vi "graph difference.vi"() -> ()   [LabVIEW 2023]
uses:
  <vilib>/addons/control/pid/autopid.llb/PID autotuning parameters (adv).ctl
  <vilib>/express/express analysis/Spectral/Block/exnSpectralBlock spectral measurements RMS poly.vi
  <vilib>/express/express analysis/Spectral/Block/exnSpectralBlock spectral measurements RMS DDT.vi
  <vilib>/express/express analysis/Spectral/XNode/ExpressSpectralMeasurementsBlockNode.xnode
  <vilib>/measure/NI_MABase.lvlib
  <vilib>/addons/control/pid/NI_PID_autopid.lvlib
panel:
  out "Control":waveform(dbl)(graph)
  in  "Target Frequency":dbl=10.0 caption="Frequency"
  out "tuning completed?":bool
  out "tuned PID gains":T1={"proportional gain (Kc)"=1.0, "integral time (Ti, min)"=0.01, "derivative time (Td, min)"=0.0} {"derivative time (Td, min)" format="%#.6g"; "integral time (Ti, min)" format="%#.6g"; "proportional gain (Kc)" format="%#.6g"}
  in  "Autotune Control":bool
  out "Backward 2":bool
  out "Forward 2":bool
  out "dt":dbl
  out "Target Waveform Graph":dynamicdata(graph)
  out "Fast Fourier Transform Target":dynamicdata(graph)
  out "Frequency Control Array":dbl[](array[numeric])
  in  "Frequency Control":dbl
  in  "amplitude 2":dbl=1.0 format="%0.2p"
  out "Phase 2":dbl
  in  "Frequency 2":dbl
  in  "stop 3":bool
  in  "frequency":dbl=10.0 format="%0.2p"
  out "Waveform Graph 2":waveform(dbl)(graph)
  in  "sampling info 2":cluster{"Fs":dbl, "#s":dbl}={"Fs"=1000.0, "#s"=1000.0} {"Fs" format="%.2p"}
  out "Difference Graph":dynamicdata(graph)
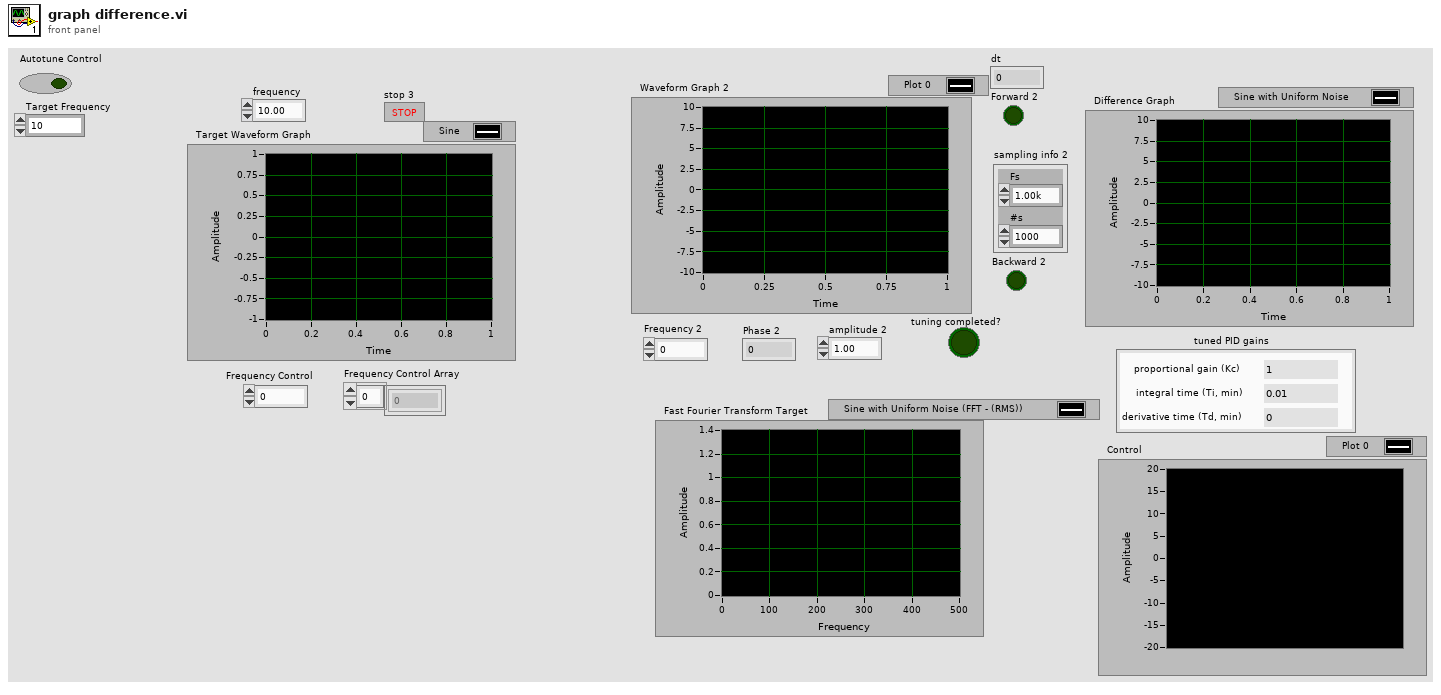
[diagram p1: front panel]
types:
  T1 = cluster{"proportional gain (Kc)":dbl, "integral time (Ti, min)":dbl, "derivative time (Td, min)":dbl}
  T2 = cluster{"averaging mode":u16, "weighting mode":u16, "number of averages":u32}
  T3 = cluster{"dB On (F)":bool, "unwrap phase (F)":bool, "convert to degree (F)":bool}
  T4 = typedef "NI_PID_autopid.lvlib/PID autotuning parameters (adv).ctl" = cluster{"technique":u16, "type of controller":u16, "control specification":u16, "amplitude":dbl}
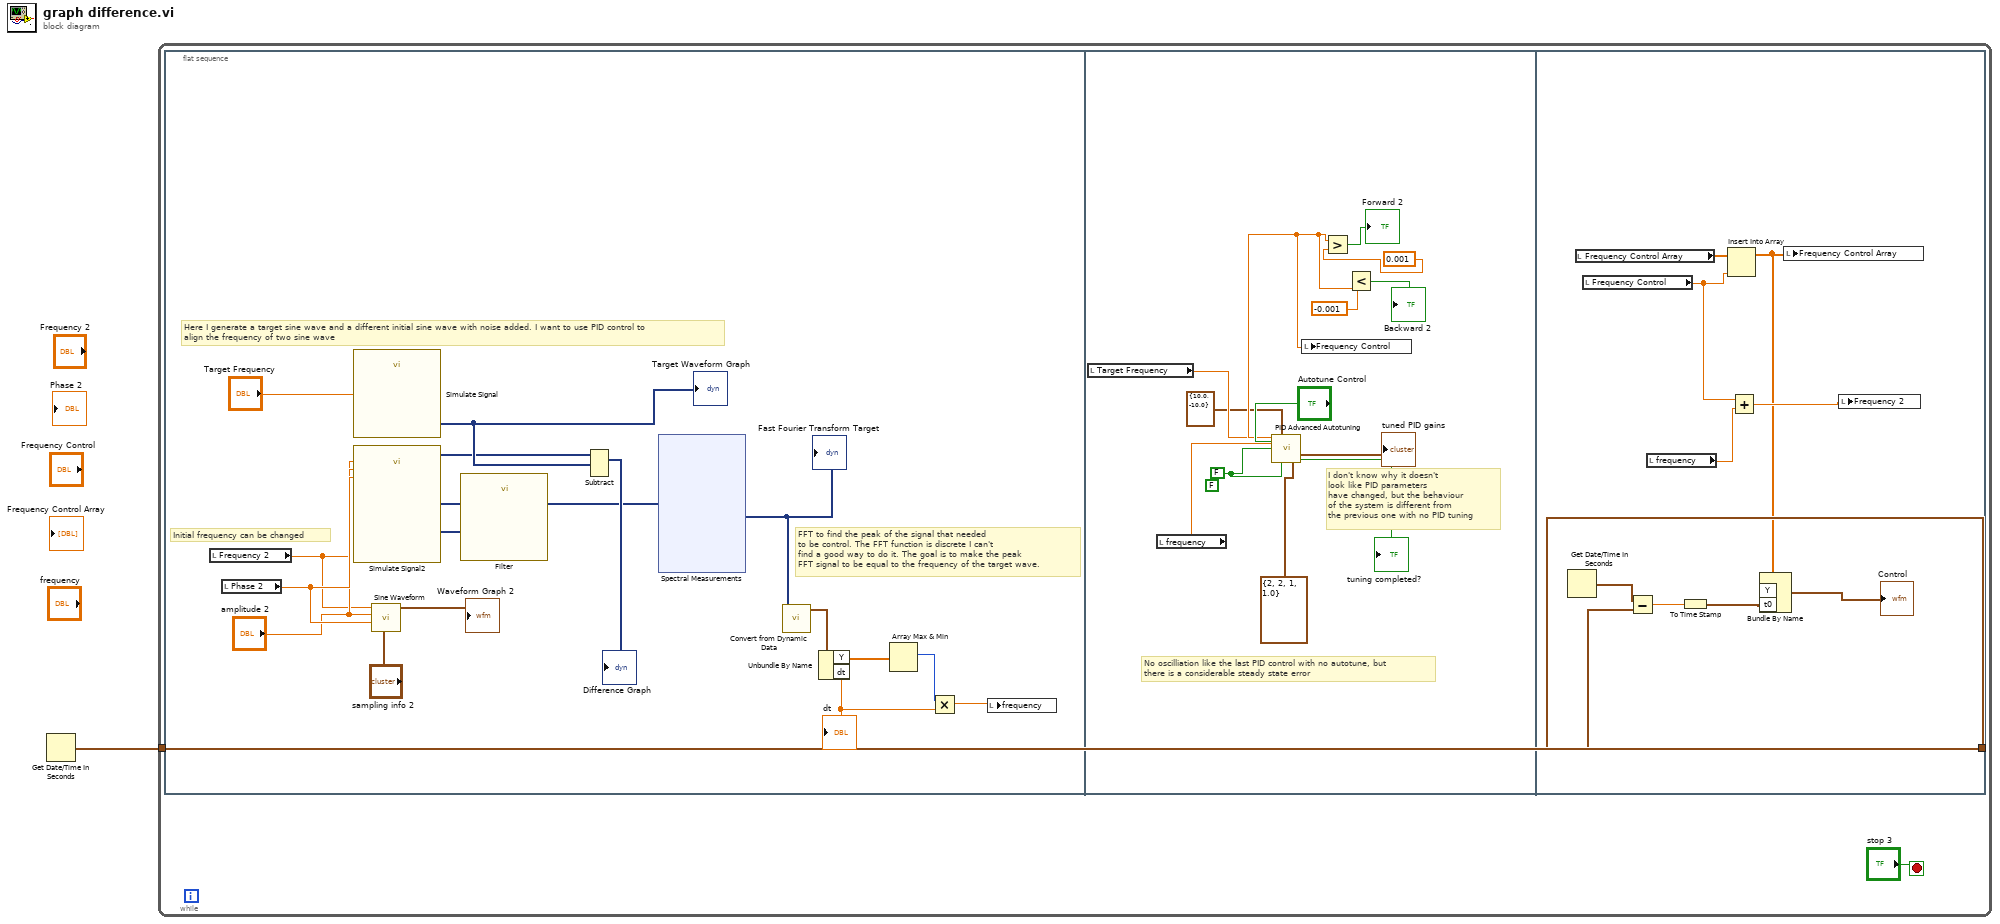
[diagram p0: block diagram]
diagram:
  n1 = Get Date/Time In Seconds() -> (seconds since 1Jan1904=w1:timestamp)
  n2 = while {
    tunnel: w1 -> [w2]
    stop <- "stop 3" stop-if-true
    n3 = flat-sequence {
      tunnel: w2 -> [w47]
      frame #0 {
        # "Initial frequency can be changed"
        # "FFT to find the peak of the signal that needed\nto be control. The FFT function is discrete I can't \nfind a good way to do it. The goal is to make the peak\nFFT signal to be equal to the frequency of the target wave."
        # "Here I generate a target sine wave and a different initial sine wave with noise added. I want to use PID control to \nalign the frequency of two sine wave"
        n4 = local read "Frequency 2"() -> (w15:dbl)
        n5 = local read "Phase 2"() -> (w17:dbl)
        n6 = call "Simulate Signal"("Frequency"="Target Frequency") -> ("Sine"=w13:dynamicdata)  [unwired: 13 in, 1 out]
        "Target Waveform Graph" <- w13
        n7 = call "Simulate Signal2"("Frequency"=w15, "Amplitude"="amplitude 2", "Phase"=w17) -> ("Sine with Uniform Noise"=w11:dynamicdata)  [unwired: 11 in, 1 out]
        n8 = call <vilib>:"Sine Waveform.vi"("sampling info"="sampling info 2", "phase"=w17, "amplitude"="amplitude 2", "frequency"=w15) -> ("signal out"=→"Waveform Graph 2":waveform(dbl))  [unwired: 6 in, 1 out]
        n9 = call "Filter"("Signal"=w11) -> ()  [unwired: 9 in, 2 out]
        n10 = Subtract(1:w13, 2:w11) -> (0:→"Difference Graph":dynamicdata)  [unwired: 1 in, 1 out]
        n11 = xnode "Spectral Measurements"("Signals"=w11) -> ("FFT - (RMS)"=w10:dynamicdata)  [unwired: 1 in, 2 out]
        "Fast Fourier Transform Target" <- w10
        n12 = call "Convert from Dynamic Data"("Dynamic Data Type"=w10) -> ("Waveform"=w9:waveform(dbl))  [unwired: 3 in]
        n13 = Unbundle By Name(w9) -> ("Y"=w8:dbl[], "dt"=w6:dbl)
        "dt" <- w6
        n14 = Array Max & Min(array=w8) -> (max index (indices)=w7:i32)  [unwired: 3 out]
        n15 = Multiply(x=w7, y=w6) -> (x*y=w5:dbl)
        n16 = local write "frequency"(w5) -> ()
      }
      frame #1 {
        (unwired) FALSE ("reinitialize? (F)")
        w30 = FALSE ("reinitialize? (F)")
        # "I don't know why it doesn't \nlook like PID parameters \nhave changed, but the behaviour \nof the system is different from \nthe previous one with no PID tuning"
        # "No oscilliation like the last PID control with no autotune, but \nthere is a considerable steady state error"
        n17 = local read "Target Frequency"() -> (w36:dbl)
        n18 = local read "frequency"() -> (w37:dbl)
        n19 = call <vilib>:"PID Advanced Autotuning.vi"("setpoint"=w36, "output range"=cluster{"output high":dbl, "output low":dbl} {"output high"=10.0, "output low"=-10.0}, "auto? (F)"="Autotune Control", "process variable"=w37, "autotune? (F)"=w30, "reinitialize? (F)"=w30, "autotuning parameters"=T4 {"technique"=2, "type of controller"=2, "control specification"=1, "amplitude"=1.0}) -> ("output"=w38:dbl, "tuned PID gains"=→"tuned PID gains":T1, "tuning completed?"=→"tuning completed?":bool)  [unwired: 6 in]
        n20 = local write "Frequency Control"(w38) -> ()
        n21 = Greater?(x=w38, y=0.001) -> (0:→"Forward 2":bool)
        n22 = Less?(x=w38, y=-0.001) -> (x < y?=→"Backward 2":bool)
      }
      frame #2 {
        n23 = Get Date/Time In Seconds() -> (seconds since 1Jan1904=w48:timestamp)
        n24 = local read "Frequency Control Array"() -> (w51:dbl[])
        n25 = local read "Frequency Control"() -> (w49:dbl)
        n26 = Subtract(x=w48, y=w47) -> (x-y=w46:dbl)
        n27 = local read "frequency"() -> (w50:dbl)
        n28 = To Time Stamp(1:w46) -> (0:w44:timestamp)
        n29 = Insert Into Array(array=w51, new element=w49) -> (w42:dbl[])  [unwired: 1 in]
        n30 = Add(x=w49, y=w50) -> (x+y=w43:dbl)
        n31 = Bundle By Name("Y"=w42, "t0"=w44) -> (→"Control":waveform(dbl))  [unwired: 1 in]
        n32 = local write "Frequency Control Array"(w42) -> ()
        n33 = local write "Frequency 2"(w43) -> ()
      }
    }
  }
